vi "Set Ramp Rates.vi"(0 "Y-Axis Communications Config":T1={"GPIB address"=22, "GPIB bus"=0, "connection ID"=refnum, "IP"="192.168.2.200", "Active Comm Interface"=0, "Serial Port"="", "Programmer Type"=0} {"Programmer Type" items=["Model 430", "Model 420"]; "Active Comm Interface" items=["TCP/IP (Model 430 Only)", "RS232", "IEEE488"]}, 1 "Y Rate (T/min)":dbl format="%#_13g", 4 "Z-Axis Communications Config":T1={"GPIB address"=22, "GPIB bus"=0, "connection ID"=refnum, "IP"="192.168.2.200", "Active Comm Interface"=0, "Serial Port"="", "Programmer Type"=0} {"Programmer Type" items=["Model 430", "Model 420"]; "Active Comm Interface" items=["TCP/IP (Model 430 Only)", "RS232", "IEEE488"]}, 5 "Z Rate (T/min)":dbl format="%#_13g", 11 "error in":T2) -> (14 "within limits?":bool=TRUE, 18 "error out":T2)   [LabVIEW 2016]
uses:
  Instrument_Setup.vi
panel:
  out "Z-Const":dbl format="%#_13g"
  out "Y-Const":dbl format="%#_13g"
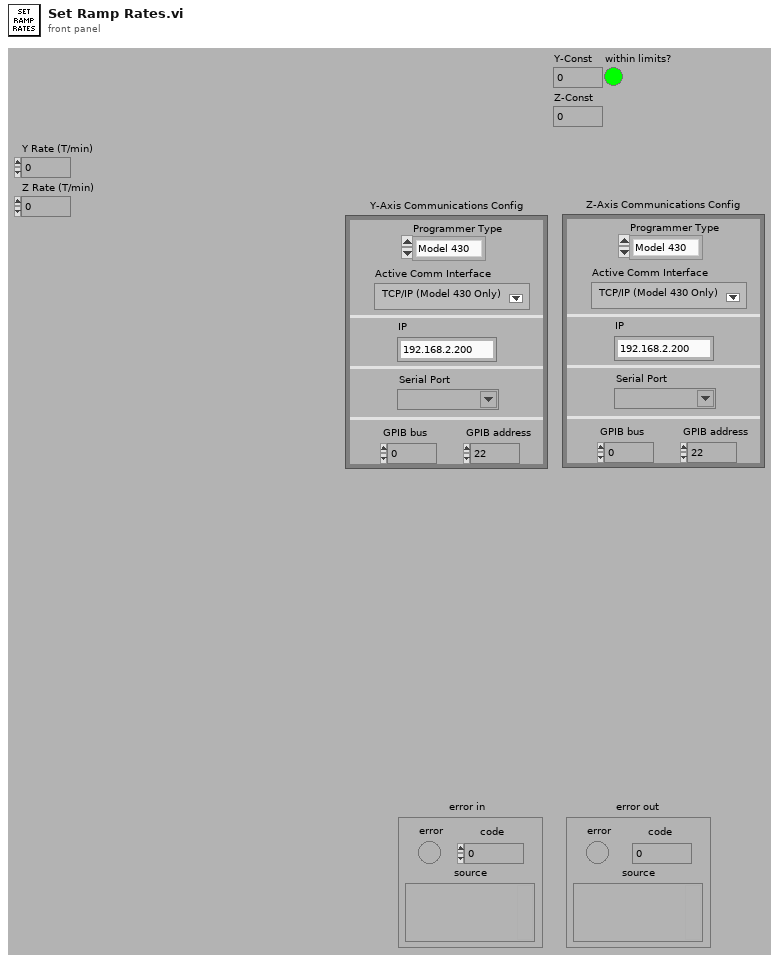
[diagram p1: front panel]
types:
  T1 = cluster{"GPIB address":i16, "GPIB bus":i16, "connection ID":refnum<k5>, "IP":string, "Active Comm Interface":u16, "Serial Port":refnum<visa-resource-name>, "Programmer Type":u16}
  T2 = cluster{"error":bool, "code":i32, "source":string}
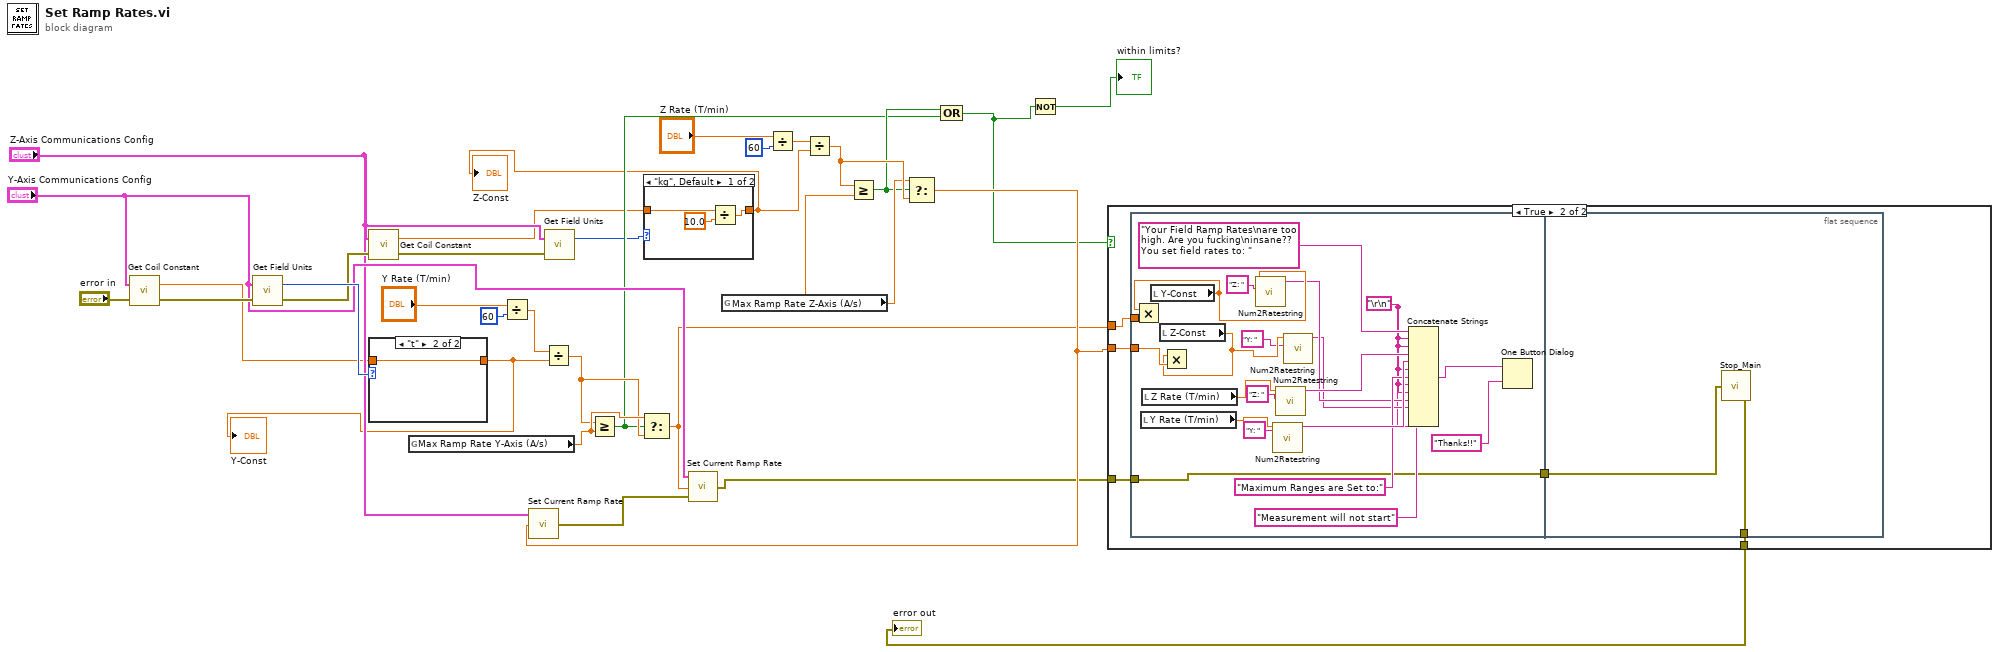
[diagram p0: block diagram]
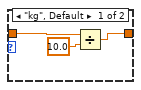
[diagram p4: hidden frame]
diagram:
  n1 = call "Get Coil Constant.vi"("error in"="error in", "Communications Config"="Y-Axis Communications Config") -> ("error out"=w30:T2, "Coil Constant"=w9:dbl)
  n2 = call "Get Field Units.vi"("error in"=w30, "Z-Axis Communications Config"="Y-Axis Communications Config") -> ("error out"=w28:T2, "Field Units"=w31:enum16{"kg", "t"})
  n3 = call "Get Coil Constant.vi"("error in"=w28, "Communications Config"="Z-Axis Communications Config") -> ("error out"=w29:T2, "Coil Constant"=w8:dbl)
  n4 = case shown="\"t\"" w31 {
    tunnel: w9 -> [w34 w35]
    tunnel: [w33 w35] -> w7
    frame "kg", Default {
      n5 = Divide(x=w34, y=10.0) -> (x/y=w33:dbl)
    }
    frame "t" {
    }
  }
  "Y-Const" <- w7
  n6 = global read "Instrument_Setup.vi" "Max Ramp Rate Y-Axis (A/s)"() -> (w17:dbl)
  n7 = Divide(x="Y Rate (T/min)", y=60) -> (x/y=w20:dbl)
  n8 = Divide(x=w20, y=w7) -> (x/y=w16:dbl)
  n9 = call "Get Field Units.vi"("error in"=w29, "Z-Axis Communications Config"="Z-Axis Communications Config") -> ("Field Units"=w5:enum16{"kg", "t"})  [unwired: 1 out]
  n10 = Greater Or Equal?(x=w16, y=w17) -> (x >= y?=w12:bool)
  n11 = Select(t=w17, s=w12, f=w16) -> (s? t:f=w10:dbl)
  n12 = case shown="\"kg\", Default" w5 {
    tunnel: w8 -> [w38 w39]
    tunnel: [w37 w39] -> w6
    frame "kg", Default {
      n13 = Divide(x=w38, y=10.0) -> (x/y=w37:dbl)
    }
    frame "t" {
    }
  }
  "Z-Const" <- w6
  n14 = global read "Instrument_Setup.vi" "Max Ramp Rate Z-Axis (A/s)"() -> (w14:dbl)
  n15 = Divide(x="Z Rate (T/min)", y=60) -> (x/y=w19:dbl)
  n16 = Divide(x=w19, y=w6) -> (x/y=w15:dbl)
  n17 = Greater Or Equal?(x=w15, y=w14) -> (x >= y?=w13:bool)
  n18 = Select(t=w14, s=w13, f=w15) -> (s? t:f=w11:dbl)
  n19 = call "Set Current Ramp Rate.vi"("Communications Config"="Z-Axis Communications Config", "Ramp Rate (A/sec)"=w11) -> ("error out"=w18:T2)  [unwired: 3 in]
  n20 = call "Set Current Ramp Rate.vi"("Communications Config"="Y-Axis Communications Config", "Ramp Rate (A/sec)"=w10, "error in"=w18) -> ("error out"=w2:T2)  [unwired: 2 in]
  n21 = Compound Arithmetic op=OR(w13, w12) -> (w4:bool)
  n22 = Not(x=w4) -> (.not. x?=→"within limits?":bool)
  n23 = case shown="True" w4 {
    tunnel: w11 -> [_ w45]
    tunnel: w10 -> [_ w44]
    tunnel: w2 -> [w40 w42]
    tunnel: [w40 w41] -> w1
    frame False {
    }
    frame True {
      n24 = flat-sequence {
        tunnel: w45 -> [w66]
        tunnel: w44 -> [w65]
        tunnel: [w46] -> w43
        tunnel: w42 -> [w46]
        tunnel: w43 -> [w68]
        tunnel: [w67] -> w41
        frame #0 {
          w51 = "\r\n"
          n25 = local read "Y Rate (T/min)"() -> (w57:dbl)
          n26 = local read "Z Rate (T/min)"() -> (w58:dbl)
          n27 = local read "Y-Const"() -> (w60:dbl)
          n28 = Multiply(x=w60, y=w65) -> ()  [unwired: 1 out]
          n29 = local read "Z-Const"() -> (w59:dbl)
          n30 = Multiply(x=w59, y=w66) -> ()  [unwired: 1 out]
          n31 = call "Num2Ratestring.vi"("String"="Z: ", "In"=w60) -> ("Out"=w53:string)  [unwired: 9 in]
          n32 = call "Num2Ratestring.vi"("String"="Y: ", "In"=w57) -> ("Out"=w55:string)  [unwired: 9 in]
          n33 = call "Num2Ratestring.vi"("String"="Z: ", "In"=w58) -> ("Out"=w56:string)  [unwired: 9 in]
          n34 = call "Num2Ratestring.vi"("String"="Y: ", "In"=w59) -> ("Out"=w52:string)  [unwired: 9 in]
          n35 = Concatenate Strings("Your Field Ramp Rates\nare too high. Are you fucking\ninsane?? You set field rates to: ", w51, w51, w56, w55, w51, "Maximum Ranges are Set to:", w51, w51, w53, w52, w51, "Measurement will not start") -> (w63:string)
          n36 = One Button Dialog(message=w63, button name ("OK")="Thanks!!") -> ()  [unwired: 1 out]
        }
        frame #1 {
          n37 = call "Stop_Main.vi"("error in"=w68) -> ("error out"=w67:errorcluster)
        }
      }
    }
  }
  "error out" <- w1
